vi "Add New Landmarks.vi"(8 "error in (no error)":errorcluster, 10 "SLAM In":T1, 11 "New LM's":T3(array[cluster])) -> (0 "error out":errorcluster, 2 "SLAM Out":T1)   [LabVIEW 2009]
uses:
  Controls/SLAM.ctl
  <vilib>/Analysis/Matrix/Datatypes/RealMatrix.ctl
  <vilib>/Analysis/Matrix/NI_Matrix.lvlib
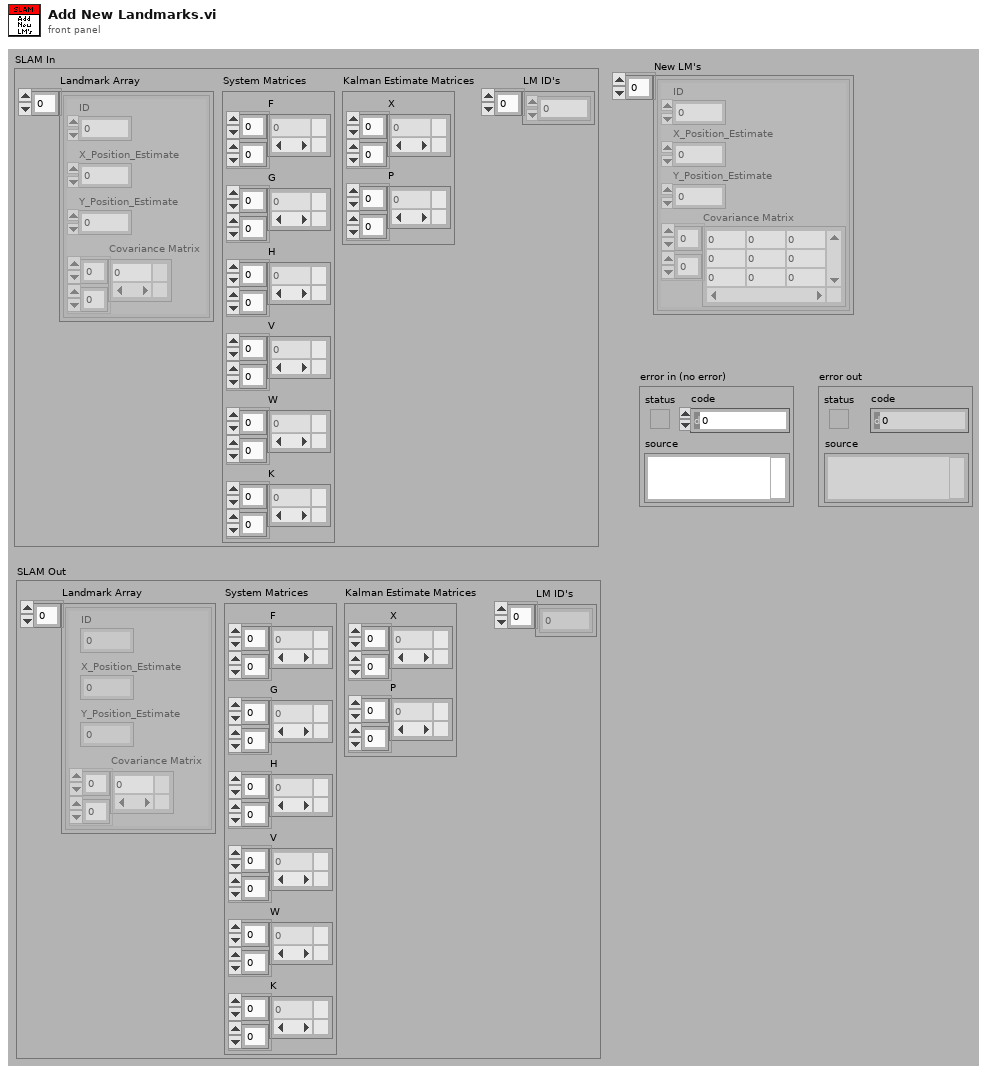
[diagram p1: front panel]
types:
  T1 = typedef "SLAM.ctl" = cluster{"Landmark Array":cluster{"ID":dbl, "X_Position_Estimate":dbl, "Y_Position_Estimate":dbl, "Covariance Matrix":T2}[], "System Matrices":cluster{"F":T2, "G":T2, "H":T2, "V":T2, "W":T2, "K":T2}, "Kalman Estimate Matrices":cluster{"X":T2, "P":T2}, "LM ID's":dbl[]}
  T2 = typedef "NI_Matrix.lvlib/RealMatrix.ctl" = dbl[][]
  T3 = cluster{"ID":dbl, "X_Position_Estimate":dbl, "Y_Position_Estimate":dbl, "Covariance Matrix":T2}[]
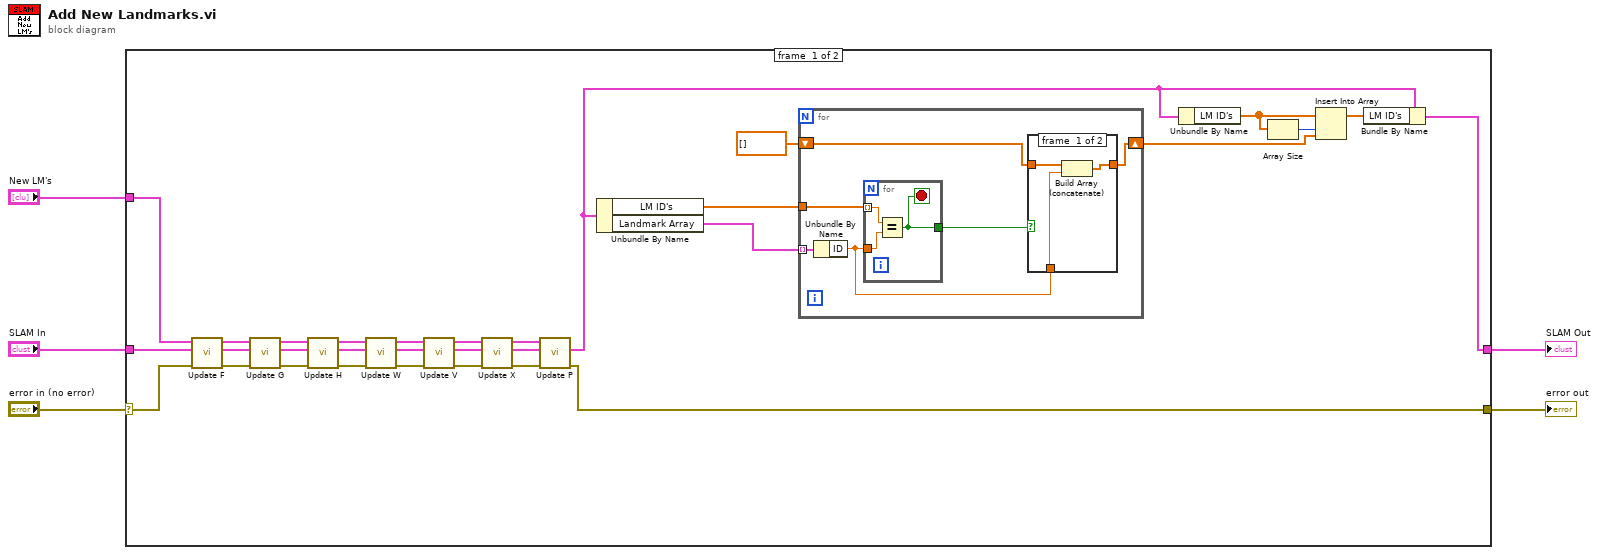
[diagram p0: block diagram]
diagram:
  n1 = case shown="No Error" "error in (no error)" {
    selector: "error in (no error)" -> [w15 w51]
    tunnel: "SLAM In" -> [w36 w50]
    tunnel: "New LM's" -> [w35 _]
    tunnel: [w6 w50] -> w3
    tunnel: [w16 w51] -> w2
    frame #0 {
      n2 = call "Update F.vi"("error in (no error)"=w15, "SLAM In"=w36, "New LM's In"=w35) -> ("error out"=w34:errorcluster, "SLAM Out"=w33:T1, "New LM's Out"=w32:T3)  [unwired: 6 in]
      n3 = call "Update G.vi"("error in (no error)"=w34, "SLAM In"=w33, "New LM's In"=w32) -> ("error out"=w31:errorcluster, "SLAM Out"=w30:T1, "New LM's Out"=w29:T3)  [unwired: 6 in]
      n4 = call "Update H.vi"("error in (no error)"=w31, "SLAM In"=w30, "New LM's In"=w29) -> ("error out"=w28:errorcluster, "SLAM Out"=w27:T1, "New LM's Out"=w26:T3)  [unwired: 6 in]
      n5 = call "Update W.vi"("error in (no error)"=w28, "SLAM In"=w27, "New LM's In"=w26) -> ("error out"=w25:errorcluster, "SLAM Out"=w23:T1, "New LM's Out"=w24:T3)  [unwired: 6 in]
      n6 = call "Update V.vi"("error in (no error)"=w25, "SLAM In"=w23, "New LM's In"=w24) -> ("error out"=w22:errorcluster, "SLAM Out"=w20:T1, "New LM's Out"=w21:T3)  [unwired: 6 in]
      n7 = call "Update X.vi"("error in (no error)"=w22, "SLAM In"=w20, "New LM's In"=w21) -> ("error out"=w19:errorcluster, "SLAM Out"=w18:T1, "New LM's Out"=w17:T3)  [unwired: 6 in]
      n8 = call "Update P.vi"("error in (no error)"=w19, "SLAM In"=w18, "New LM's In"=w17) -> ("error out"=w16:errorcluster, "SLAM Out"=w8:T1)  [unwired: 6 in, 1 out]
      n9 = Unbundle By Name(w8) -> ("LM ID's"=w10:dbl[], "Landmark Array"=w9:T3)
      n10 = for {
        tunnel: w10 -> [w38]
        tunnel: w9 -> [w42] mode=indexing
        shift-right: [w40] -> w14
        shift-left: dbl[] [] -> [w41]
        n11 = Unbundle By Name(w42) -> ("ID"=w39:dbl)
        n12 = for {
          tunnel: w38 -> [w49] mode=indexing
          tunnel: w39 -> [w47]
          tunnel: [w48] -> w37
          stop <- w48 stop-if-true
          n13 = Equal?(x=w49, y=w47) -> (x = y?=w48:bool)
        }
        n14 = case shown="True" w37 {
          tunnel: w41 -> [w45 w46]
          tunnel: w39 -> [w44 _]
          tunnel: [w43 w46] -> w40
          frame #0 {
            n15 = Build Array (concatenate)(w45, w44) -> (w43:dbl[])
          }
          frame #1 {
          }
        }
      }
      n16 = Unbundle By Name(w8) -> ("LM ID's"=w12:dbl[])
      n17 = Array Size(array=w12) -> (size(s)=w13:i32)
      n18 = Insert Into Array(array=w12, index=w13, new element=w14) -> (w7:dbl[])
      n19 = Bundle By Name(cluster=w8, "LM ID's"=w7) -> (w6:T1)
    }
    frame #1 {
    }
  }
  "error out" <- w2
  "SLAM Out" <- w3
